vi "PluginsLoaderService_Create.vi"(8 "error in (no error)":errorcluster) -> (0 "error out":errorcluster, 1 "AvailablePluginsEvent":refnum<user-event>, 2 "Commander":refnum<class "PluginsLoaderCommander.lvclass">, 3 "PluginsLoaderService out":refnum<class "PluginsLoaderService.lvclass">)   [LabVIEW 2014, in "PluginsThread.lvlib" / "PluginsLoaderService.lvclass"]
uses:
  PluginsLoaderService.lvclass
  _Plugins/GCMPlugin/GCMPlugin.lvclass
  PluginsLoaderCommander/PluginsLoaderCommander.lvclass
  PluginsLoaderService.lvclass/PluginsLoaderService.ctl
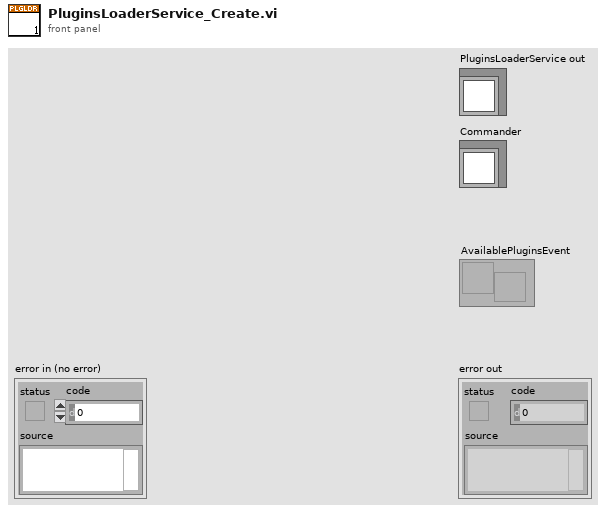
[diagram p1: front panel]
types:
  T1 = cluster{"CurrentItem":refnum<vi>, "AvailablePlugins":refnum<class "GCMPlugin.lvclass">[]}
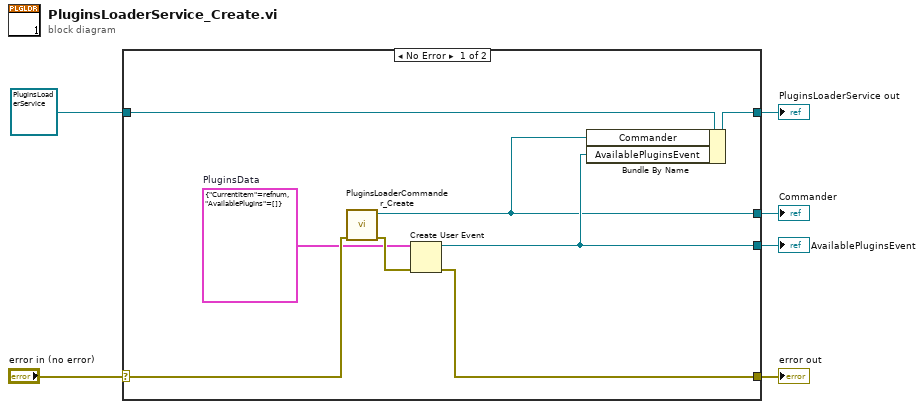
[diagram p0: block diagram]
diagram:
  n1 = case shown="No Error" "error in (no error)" {
    selector: "error in (no error)" -> [w12 w16]
    tunnel: [w8 w16] -> w5
    tunnel: [w13 w15] -> w3
    tunnel: refnum<class "PluginsLoaderService.lvclass"> refnum ("PluginsLoaderService in") -> [w14 w15]
    tunnel: [w9 _] -> w2
    tunnel: [w7 _] -> w1
    frame No Error {
      w10 = T1 {"CurrentItem"=refnum, "AvailablePlugins"=[]}  # PluginsData
      n2 = call "PluginsLoaderCommander_Create.vi"("error in (no error)"=w12) -> ("error out"=w11:errorcluster, "PluginsLoaderCommander out"=w7:refnum<class "PluginsLoaderCommander.lvclass">)  [unwired: 9 in]
      n3 = Create User Event(user event datatype=w10, error in=w11) -> (user event=w9:refnum<user-event>, error out=w8:errorcluster)
      n4 = Bundle By Name(cluster=w14, "Commander"=w7, "AvailablePluginsEvent"=w9) -> (w13:refnum<class "PluginsLoaderService.lvclass">)
    }
    frame Error {
    }
  }
  "error out" <- w5
  "PluginsLoaderService out" <- w3
  "AvailablePluginsEvent" <- w2
  "Commander" <- w1
